vi "RW_LIR.vi"(7 "N_moduls":i32, 8 "error in":errorcluster, 9 "Param Referense":T1, 10 "Data Reference":T2, 11 "Status Reference":T3) -> (0 "error out":errorcluster, 1 "stopped":bool)   [LabVIEW 2019]
uses:
  projects/Graphetron_1/Batcher/GM2_2/az_parameters_200121.vi
  Modbus/MB_TCP3/ICPCON ET-7018/ICPCON ET-7018.lvclass
  Modbus/MB_TCP3/ICPCON ET-7016/ICPCON ET-7016.lvclass
  Modbus/MB_TCP3/ICPCON ET-7051/ICPCON ET-7051.lvclass
  Modbus/MB_TCP3/ICPCON ET-7017/ICPCON ET-7017.lvclass
  Modbus/MB_TCP3/ICPCON ET-7018i/ICPCON ET-7018i.lvclass
  Modbus/MB_TCP3/ICPCON ET-7024i/ICPCON ET-7024i.lvclass
  Modbus/MB_TCP3/ZERO/ZERO.lvclass
  Modbus/MB_TCP3/NS300/NS300.lvclass
  Modbus/MB_TCP3/ICPCON ET-7042i/ICPCON ET-7042i.lvclass
  Modbus/MB_TCP3/MB_TCP.lvclass
  Modbus/MB_TCP3/MB timeouts.ctl
  Modbus/NI_modbus_upd/TCP/tcp timeouts.ctl
  Modbus/NI_modbus_upd/TCP/TCP.lvclass
  Modbus/ICPCON Param/ICPCON_Param.lvlib
  Modbus/MB_TCP3/Execute.vi
  Modbus/MB_TCP3/LIR-919D/LIR-919D.lvclass
  D:/my_projects/projects/Algorithms/Labview/19/Modbus/MB_TCP2/MB_TCP.lvclass
  Modbus/ICPCON Status/Ctl/ICPCON Status.ctl
  Modbus/ICPCON Registers/Ctl/ICPCON Data.ctl
  Modbus/ICPCON Registers/ICPCON Registers.lvlib
  Modbus/ICPCON Param/ICPCON Param.ctl
  Modbus/MB_TCP3/Eth timeouts.ctl
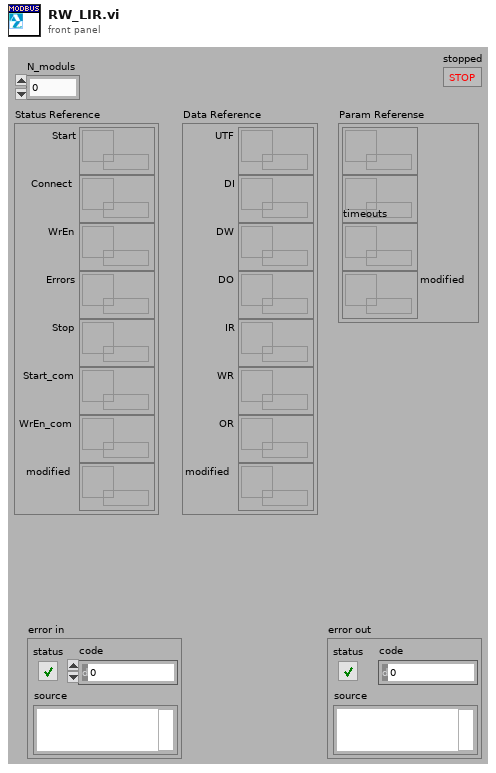
[diagram p1: front panel]
types:
  T1 = typedef "ICPCON_Param.lvlib/ICPCON Param.ctl" = cluster{"IP addr":refnum<data-value>, "MVIName":refnum<data-value>, "timeouts":refnum<data-value>, "modified":refnum<data-value>}
  T2 = typedef "ICPCON Registers.lvlib/ICPCON Data.ctl" = cluster{"UTF":refnum<data-value>, "DI":refnum<data-value>, "DW":refnum<data-value>, "DO":refnum<data-value>, "IR":refnum<data-value>, "WR":refnum<data-value>, "OR":refnum<data-value>, "modified":refnum<data-value>}
  T3 = typedef "ICPCON Status.lvlib/ICPCON Status.ctl" = cluster{"Start":refnum<data-value>, "Connect":refnum<data-value>, "WrEn":refnum<data-value>, "Errors":refnum<data-value>, "Stop":refnum<data-value>, "Start_com":refnum<data-value>, "WrEn_com":refnum<data-value>, "modified":refnum<data-value>}
  T4 = enum16{"initialize", "call modules", "work", "stop modules", "standby"}
  T5 = typedef "TCP.lvclass/tcp timeouts.ctl" = cluster{"connect timeout":i32, "write timeout":i32, "read timeout":i32}
  T6 = typedef "MB_TCP.lvclass/MB timeouts.ctl" = cluster{"reconn_timeout":i32, "N attempt max":i32, "t_reset_TTL":i32, "period":i32}
  T7 = typedef "MB_TCP.lvclass/Eth timeouts.ctl" = cluster{"conn_timeout":i32, "reconn_timeout":i32, "N attempt max":i32, "t_reset_TTL":i32, "write_timeout":i32, "read_timeout":i32, "period":i32}
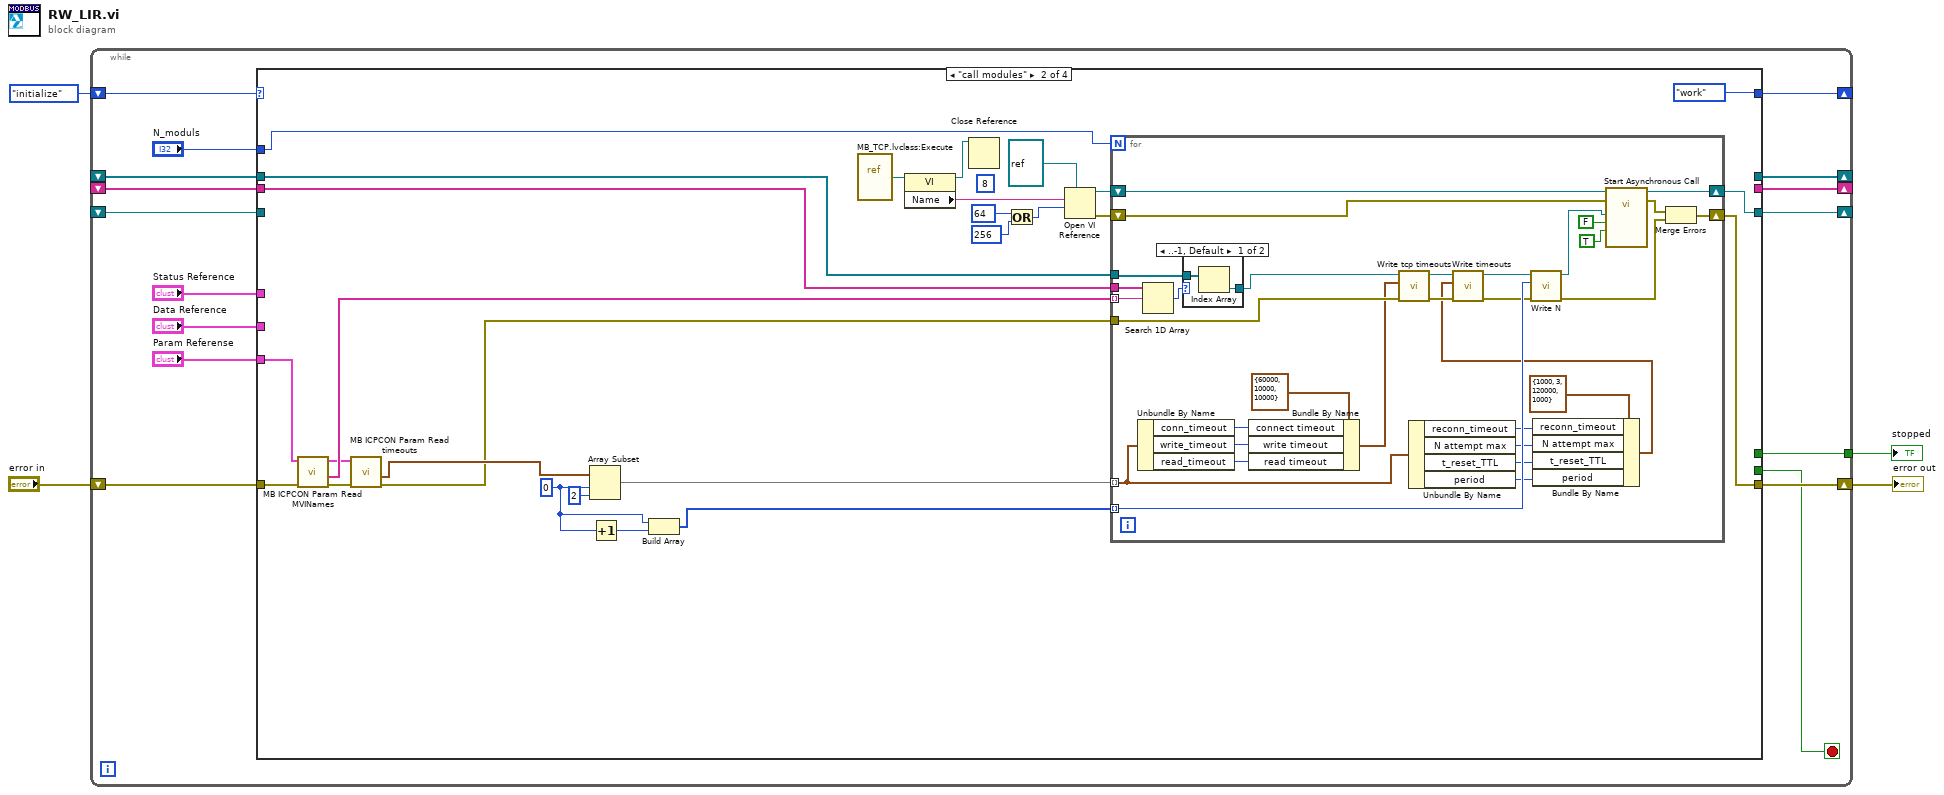
[diagram p0: block diagram]
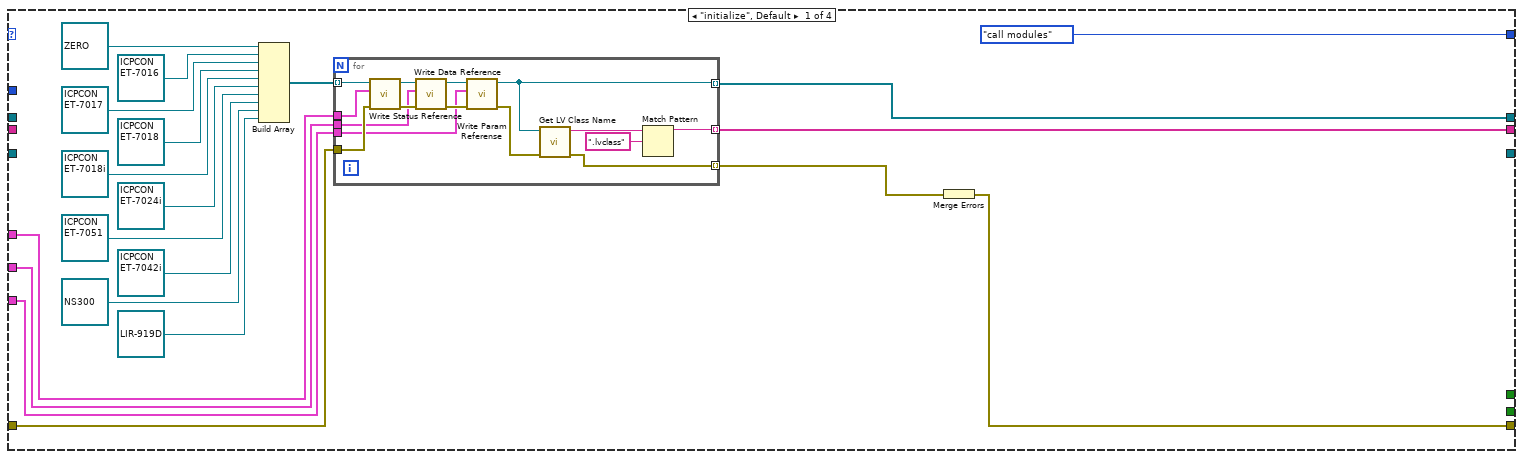
[diagram p2: hidden frame]
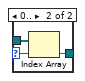
[diagram p3: hidden frame]
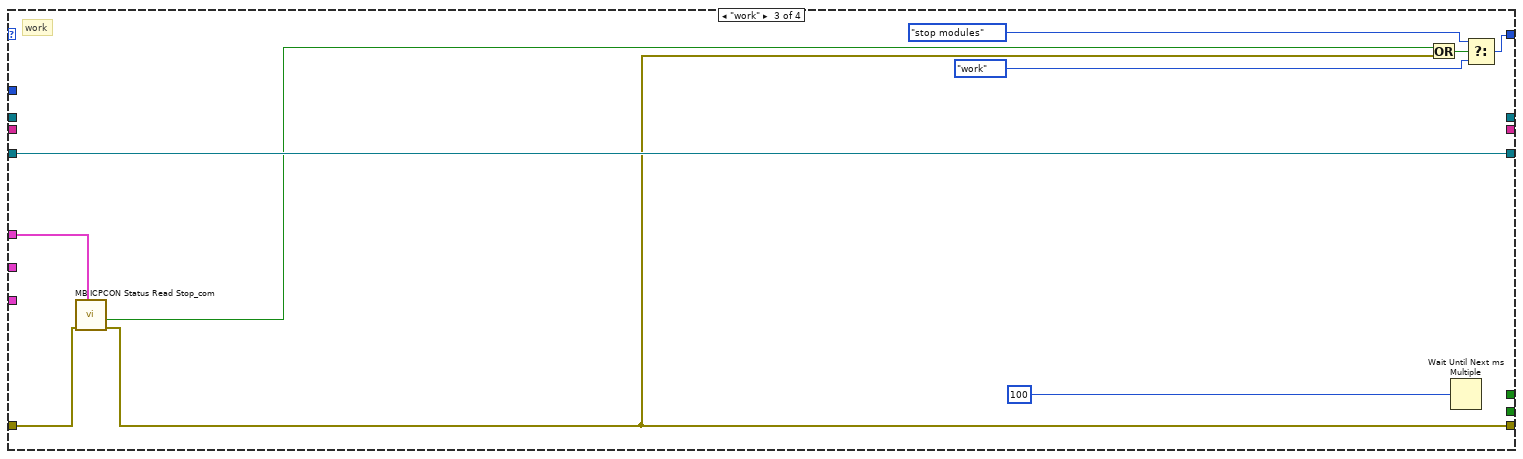
[diagram p4: hidden frame]
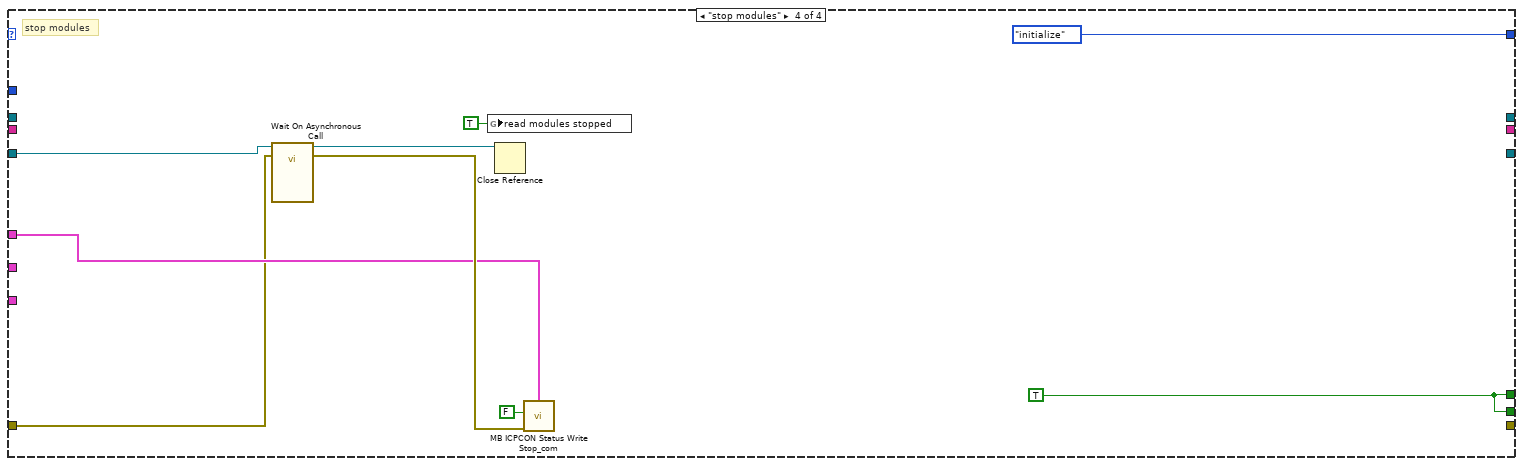
[diagram p5: hidden frame]
diagram:
  n1 = while {
    shift-right: [w20] -> _
    shift-left: T4."initialize" ("Enum") -> [w17]
    shift-right: [w16] -> w3
    shift-left: "error in" -> [w15]
    tunnel: [w14] -> w2
    shift-right: [w12] -> _
    shift-left: _ -> [w11]
    shift-right: [w10] -> _
    shift-left: _ -> [w9]
    shift-right: [w6] -> _
    shift-left: _ -> [w5]
    stop <- w13 stop-if-true
    n2 = case shown="\"call modules\"" w17 {
      tunnel: [T4."call modules" ("Enum") T4."work" ("Enum") w129 T4."initialize" ("Enum")] -> w20
      tunnel: "N_moduls" -> [_ w60 _ _]
      tunnel: "Status Reference" -> [w25 _ w122 w132]
      tunnel: [w39 w82 w121 _] -> w16
      tunnel: w15 -> [w30 w69 w123 w130]
      tunnel: [_ _ _ w138] -> w14
      tunnel: [_ _ _ w138] -> w13
      tunnel: [w38 _ _ _] -> w12
      tunnel: w11 -> [_ w59 _ _]
      tunnel: [w21 _ _ _] -> w10
      tunnel: w9 -> [_ w61 _ _]
      tunnel: "Data Reference" -> [w24 _ _ _]
      tunnel: "Param Referense" -> [w23 w57 _ _]
      tunnel: [_ w72 w124 _] -> w6
      tunnel: w5 -> [_ _ w124 w136]
      frame "initialize", Default {
        n3 = Build Array(refnum<class "ZERO.lvclass"> refnum ("ZERO.lvclass"), refnum<class "ICPCON ET-7016.lvclass"> refnum ("ICPCON ET-7016.lvclass"), refnum<class "ICPCON ET-7017.lvclass"> refnum ("ICPCON ET-7017.lvclass"), refnum<class "ICPCON ET-7018.lvclass"> refnum ("ICPCON ET-7018 in"), refnum<class "ICPCON ET-7018i.lvclass"> refnum ("ICPCON ET-7018i.lvclass"), refnum<class "ICPCON ET-7024i.lvclass"> refnum ("ICPCON ET-7024i.lvclass"), refnum<class "ICPCON ET-7051.lvclass"> refnum ("ICPCON ET-7051.lvclass"), refnum<class "ICPCON ET-7042i.lvclass"> refnum ("ICPCON ET-7042i.lvclass"), refnum<class "NS300.lvclass"> refnum ("NS300.lvclass"), refnum<class "LIR-919D.lvclass"> refnum ("LIR-919D.lvclass")) -> (w22:refnum<class "MB_TCP.lvclass">[])
        n4 = for {
          tunnel: w22 -> [w48] mode=indexing
          tunnel: [w52] -> w38 mode=indexing
          tunnel: [w55] -> w40 mode=indexing
          tunnel: w30 -> [w47]
          tunnel: w25 -> [w44]
          tunnel: w24 -> [w43]
          tunnel: w23 -> [w42]
          tunnel: [w41] -> w21 mode=indexing
          n5 = call "Write Status Reference.vi"("error in (no error)"=w47, "Status"=w44, "MB_TCP in"=w48) -> ("error out"=w46:errorcluster, "MB_TCP out"=w49:refnum<class "MB_TCP.lvclass">)  [unwired: 7 in]
          n6 = call "Write Data Reference.vi"("error in (no error)"=w46, "Data"=w43, "MB_TCP in"=w49) -> ("error out"=w50:errorcluster, "MB_TCP out"=w51:refnum<class "MB_TCP.lvclass">)  [unwired: 7 in]
          n7 = call "Write Param Referense.vi"("error in (no error)"=w50, "Param Referense"=w42, "MB_TCP in"=w51) -> ("error out"=w45:errorcluster, "MB_TCP out"=w41:refnum<class "MB_TCP.lvclass">)  [unwired: 7 in]
          n8 = call <vilib>:"Get LV Class Name.vi"("error in (no error)"=w45, "object"=w41) -> ("error out"=w55:errorcluster, "class name"=w54:string)  [unwired: 8 in]
          n9 = Match Pattern(string=w54, regular expression=".lvclass") -> (before substring=w52:string)  [unwired: 1 in, 3 out]
        }
        n10 = Merge Errors(w40) -> (w39:errorcluster)
      }
      frame "call modules" {
        w65 = 0 ("index")
        (unwired) 8 ("options")
        n11 = call "MB ICPCON Param Read MVINames.vi"("error in (no error)"=w69, "Param Reference in"=w57) -> ("error out"=w70:errorcluster, "MVIName"=w58:string[], "Param Reference out"=w56:T1)  [unwired: 7 in]
        n12 = call "MB ICPCON Param Read timeouts.vi"("error in (no error)"=w70, "Param Reference in"=w56) -> ("error out"=w62:errorcluster, "timeouts"=w68:T7[])  [unwired: 7 in, 1 out]
        n13 = Array Subset(array=w68, index=w65, length=2) -> (w66:T7[])
        n14 = Increment(x=w65) -> (x+1=w64:i32)
        n15 = Build Array(w65, w64) -> (w63:i32[])
        n16 = vi-ref "MB_TCP.lvclass:Execute.vi"() -> (w78:refnum<vi>)
        n17 = property class="VI"(reference=w78) -> (reference out=w71:refnum<vi>, "Name"=w76:string)  [unwired: 1 in, 1 out]
        n18 = Close Reference(reference=w71) -> ()  [unwired: 1 in, 1 out]
        n19 = Or(x=64 ("options"), y=256 ("options")) -> (x .or. y?=w75:i32)
        n20 = Open VI Reference(type specifier VI Refnum (for type only)=refnum<vi> refnum ("Ctl Refnum"), vi path=w76, options=w75) -> (vi reference=w77:refnum<vi>, error out=w80:errorcluster)  [unwired: 3 in]
        n21 = for {
          N: w60 -> [_]
          tunnel: w63 -> [w110] mode=indexing
          tunnel: w62 -> [w105]
          tunnel: w66 -> [w98] mode=indexing
          tunnel: w61 -> [w86]
          shift-right: [w114] -> w82
          shift-left: w80 -> [w113]
          shift-right: [w107] -> w72
          shift-left: w77 -> [w111]
          tunnel: w59 -> [w84]
          tunnel: w58 -> [w83] mode=indexing
          n22 = Unbundle By Name(w98) -> ("conn_timeout"=w101:i32, "write_timeout"=w100:i32, "read_timeout"=w99:i32)
          n23 = Search 1D Array(1D array=w84, element=w83) -> (index of element=w87:i32)  [unwired: 1 in]
          n24 = case shown="..-1, Default" w87 {
            selector: w87 -> [_ w117]
            tunnel: w86 -> [w116 w119]
            tunnel: [w115 w118] -> w85
            frame ..-1, Default {
              n25 = Index Array(array=w116) -> (element=w115:refnum<class "MB_TCP.lvclass">)  [unwired: 1 in]
            }
            frame 0.. {
              n26 = Index Array(array=w119, index=w117) -> (element=w118:refnum<class "MB_TCP.lvclass">)
            }
          }
          n27 = Bundle By Name(cluster=T5 {"connect timeout"=60000, "write timeout"=10000, "read timeout"=10000} ("tcp timeouts"), "connect timeout"=w101, "write timeout"=w100, "read timeout"=w99) -> (w97:T5)
          n28 = call "Write tcp timeouts.vi"("error in (no error)"=w105, "tcp timeouts"=w97, "MB_TCP in"=w85) -> ("error out"=w104:errorcluster, "MB_TCP out"=w106:refnum<class "MB_TCP.lvclass">)  [unwired: 7 in]
          n29 = Unbundle By Name(w98) -> ("reconn_timeout"=w96:i32, "N attempt max"=w95:i32, "t_reset_TTL"=w94:i32, "period"=w93:i32)
          n30 = Bundle By Name(cluster=T6 {"reconn_timeout"=1000, "N attempt max"=3, "t_reset_TTL"=120000, "period"=1000} ("MB timeouts"), "reconn_timeout"=w96, "N attempt max"=w95, "t_reset_TTL"=w94, "period"=w93) -> (w92:T6)
          n31 = call "Write timeouts.vi"("error in (no error)"=w104, "MB timeouts"=w92, "MB_TCP in"=w106) -> ("error out"=w88:errorcluster, "MB_TCP out"=w89:refnum<class "MB_TCP.lvclass">)  [unwired: 7 in]
          n32 = call "Write N.vi"("error in (no error)"=w88, "N"=w110, "MB_TCP in"=w89) -> ("error out"=w91:errorcluster, "MB_TCP out"=w109:refnum<class "MB_TCP.lvclass">)  [unwired: 7 in]
          n33 = call-by-ref "Start Asynchronous Call"(reference=w111, error in=w113, "write enable"=TRUE, "stop"=FALSE, "MB_TCP in"=w109) -> (reference out=w107:refnum<vi>, error out=w108:errorcluster)  [unwired: 6 in, 3 out]
          n34 = Merge Errors(w108, w91) -> (w114:errorcluster)
        }
      }
      frame "work" {
        # "work"
        n35 = call "MB ICPCON Status Read Stop_com.vi"("Status Reference"=w122, "error in (no error)"=w123) -> ("error out"=w121:errorcluster, "Stop"=w120:bool)  [unwired: 8 in]
        n36 = Or(x=w120, y=w121) -> (x .or. y?=w128:bool)
        n37 = Wait Until Next ms Multiple(millisecond multiple=u32 100) -> ()  [unwired: 1 out]
        n38 = Select(t=T4."stop modules" ("Enum"), s=w128, f=T4."work" ("Enum")) -> (s? t:f=w129:T4)
      }
      frame "stop modules" {
        w138 = TRUE
        # "stop modules"
        n39 = call-by-ref "Wait On Asynchronous Call"(reference=w136, error in=w130) -> (reference out=w135:refnum<vi>, error out=w133:errorcluster)  [unwired: 9 in, 3 out]
        n40 = global write "az_parameters_200121.vi" "read modules stopped"(TRUE ("read modules stopped")) -> ()
        n41 = Close Reference(reference=w135) -> ()  [unwired: 1 in, 1 out]
        n42 = call "MB ICPCON Status Write Stop_com.vi"("Status Reference"=w132, "error in (no error)"=w133, "Stop"=FALSE) -> ()  [unwired: 8 in, 1 out]
      }
    }
  }
  "error out" <- w3
  "stopped" <- w2
